vi "PrepTip - Copy.vi"() -> ()   [LabVIEW 2014]
uses:
  <userlib>/Nanonis Prog Interface V5/Nanonis Prog Interface.lvlib
panel:
  in  "Number of pulses":dbl=1.0
  in  "Pulse bias (V)":dbl=1.0
  in  "Pulse width (s)":dbl=0.1 min=0.0 max=100.0 format="%#_6p"
  in  "stop":bool
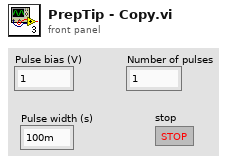
[diagram p1: front panel]
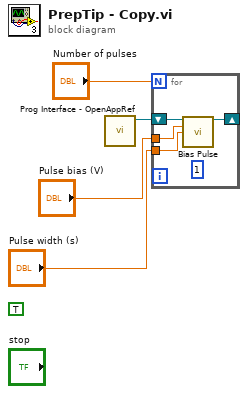
[diagram p0: block diagram]
diagram:
  (unwired) TRUE ("Wait for newest data (F=False)")
  n1 = call <userlib>:"Prog Interface - OpenAppRef.vi"() -> ("Application reference"=w1:refnum<vi>)  [unwired: 6 in, 1 out]
  n2 = for {
    N: "Number of pulses" -> [_]
    tunnel: "Pulse width (s)" -> [w6]
    tunnel: "Pulse bias (V)" -> [w5]
    shift-right: [w8] -> _
    shift-left: w1 -> [w7]
    (unwired) 1
    n3 = call <userlib>:"Bias Pulse.vi"("Application ref in"=w7, "Pulse bias (V) (1)"=w5, "Pulse width (s) (100m)"=w6) -> ("Application ref out"=w8:refnum<vi>)  [unwired: 11 in, 1 out]
  }
